vi "Set Parent.vi"(8 "error in (no error)":errorcluster, 10 "parent window refnum":T1, 11 "child window refnum":T1) -> (0 "error out":errorcluster, 1 "prev parent window refnum out":T1, 2 "parent window refnum out":T1, 3 "child window refnum out":T1)   [LabVIEW 2020, in "MacroAssert.lvlib" / "Win Util.lvlib"]
uses:
  Win Util.lvlib
  user32.dll
  Window Refnum.ctl
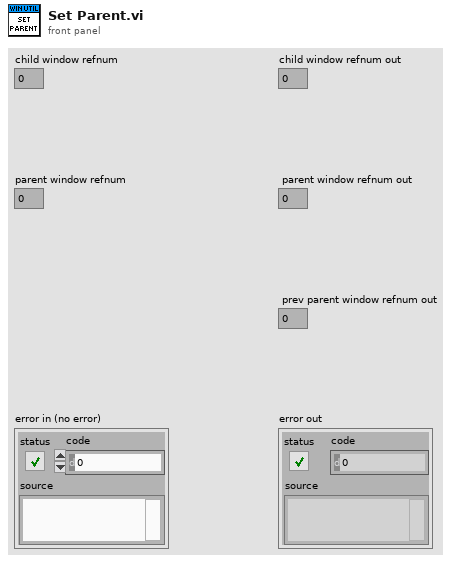
[diagram p1: front panel]
types:
  T1 = typedef "MacroAssert.lvlib/Win Util.lvlib/Window Refnum.ctl" = u64
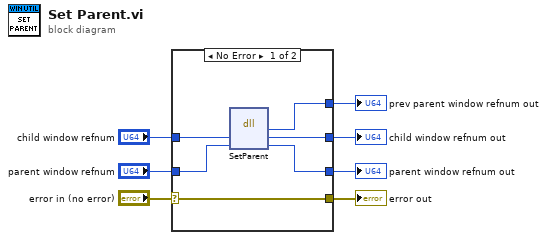
[diagram p0: block diagram]
diagram:
  n1 = case shown="No Error" "error in (no error)" {
    selector: "error in (no error)" -> [w8 w16]
    tunnel: "parent window refnum" -> [w13 w15]
    tunnel: "child window refnum" -> [w12 w14]
    tunnel: [w8 w16] -> w4
    tunnel: [w11 w15] -> w3
    tunnel: [w10 w14] -> w2
    tunnel: [w9 _] -> w1
    frame No Error {
      n2 = dll-call lib="user32.dll" fn="SetParent"("hwndChild"=w12, "hwndNewParent"=w13) -> ("return type"=w9:u64, "hwndChild"=w10:u64, "hwndNewParent"=w11:u64)  [unwired: 3 in, 2 out]
    }
    frame Error {
    }
  }
  "child window refnum out" <- w2
  "error out" <- w4
  "parent window refnum out" <- w3
  "prev parent window refnum out" <- w1
